vi "GetVoltage.vi"(4 "error in":errorcluster, 5 "connection ID":refnum<k5>) -> (0 "Voltage":string, 1 "error out":errorcluster, 2 "connection ID out":refnum<k5>, 3 "Answer":bool)   [LabVIEW 2013]
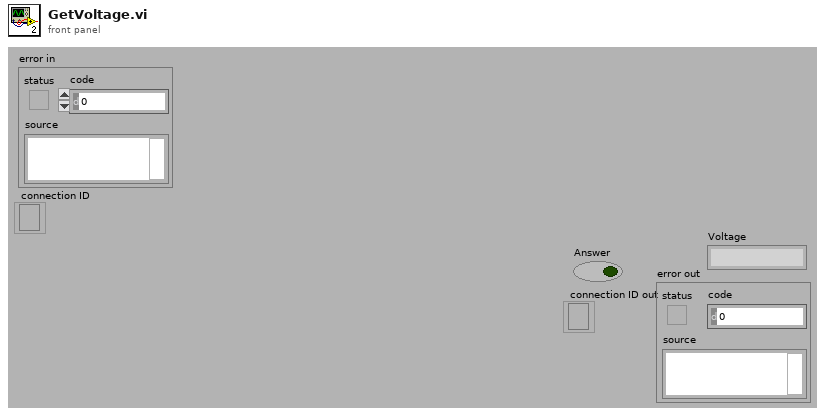
[diagram p1: front panel]
types:
  T1 = enum16{"Standard", "Buffered", "CRLF", "Immediate"}
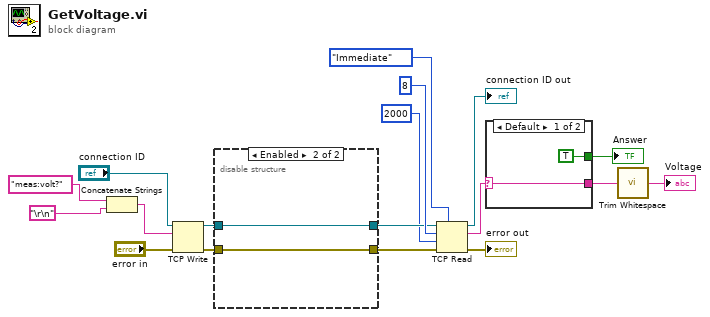
[diagram p0: block diagram]
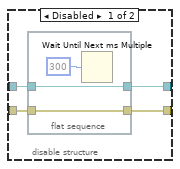
[diagram p2: hidden frame]
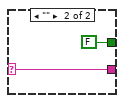
[diagram p3: hidden frame]
diagram:
  n1 = Concatenate Strings("meas:volt?" ("data in"), "\r\n") -> (w1:string)
  n2 = TCP Write(connection ID="connection ID", data in=w1, error in (no error)="error in") -> (connection ID out=w8:refnum<k5>, error out=w6:errorcluster)  [unwired: 2 out]
  n3 = disable-structure shown="Enabled" {
    disable-tunnel: w8 -> [w22 w27]
    disable-tunnel: [w21 w27] -> w7
    disable-tunnel: w6 -> [w20 w26]
    disable-tunnel: [w19 w26] -> w5
    frame Disabled {
      n4 = flat-sequence {
        tunnel: [w24] -> w21
        tunnel: w22 -> [w24]
        tunnel: w20 -> [w23]
        tunnel: [w23] -> w19
        frame #0 {
          n5 = Wait Until Next ms Multiple(millisecond multiple=u32 300) -> ()  [unwired: 1 out]
        }
      }
    }
    frame Enabled {
    }
  }
  n6 = TCP Read(connection ID=w7, bytes to read=8, error in (no error)=w5, 7:T1."Immediate" ("mode (standard)"), 9:2000 ("timeout ms (25000)")) -> (connection ID out=→"connection ID out":refnum<k5>, data out=w12:string, error out=→"error out":errorcluster)
  n7 = case shown="Default" w12 {
    selector: w12 -> [w29 w31]
    tunnel: [w29 w31] -> w17
    tunnel: [TRUE FALSE] -> w18
    frame Default {
    }
    frame "" {
    }
  }
  "Answer" <- w18
  n8 = call <vilib>:"Trim Whitespace.vi"("string"=w17) -> ("trimmed string"=→"Voltage":string)  [unwired: 1 in]
